vi "SetXMLValue.vi"(10 "Value":dbl format="%#_13g", 11 "Path":path) -> ()   [LabVIEW 2017]
uses:
  <vilib>/Utility/xml.llb/Write to XML File(string).vi
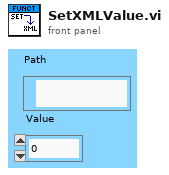
[diagram p1: front panel]
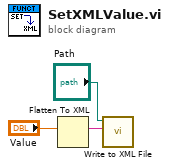
[diagram p0: block diagram]
diagram:
  n1 = Flatten To XML(anything="Value") -> (xml string=w1:string)
  n2 = call-poly <vilib>:"Write to XML File.vi"("XML Input"=w1, "XML File Path"="Path") -> ()  [unwired: 7 in, 3 out]
